vi "sick.vi"() -> ()   [LabVIEW 2014]
panel:
  out "Response":string
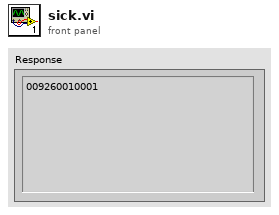
[diagram p1: front panel]
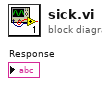
[diagram p0: block diagram]
diagram:
